vi "模拟量输入自动测试一组_fast_OK.vi"(8 "AD选择？":bool, 9 "DSP选择？":bool, 11 "第几个":i32) -> ()   [LabVIEW 2010]
uses:
  全局量/试验配置信息.vi
panel:
  in  "AD测试值":dbl[](array[numeric])
  in  "DSP测试值":dbl[](array[numeric])
  # "从0开始"
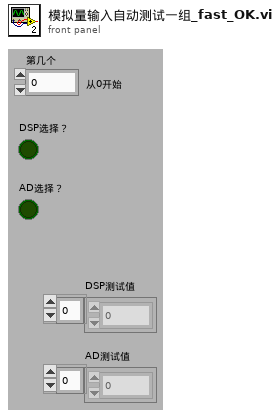
[diagram p1: front panel]
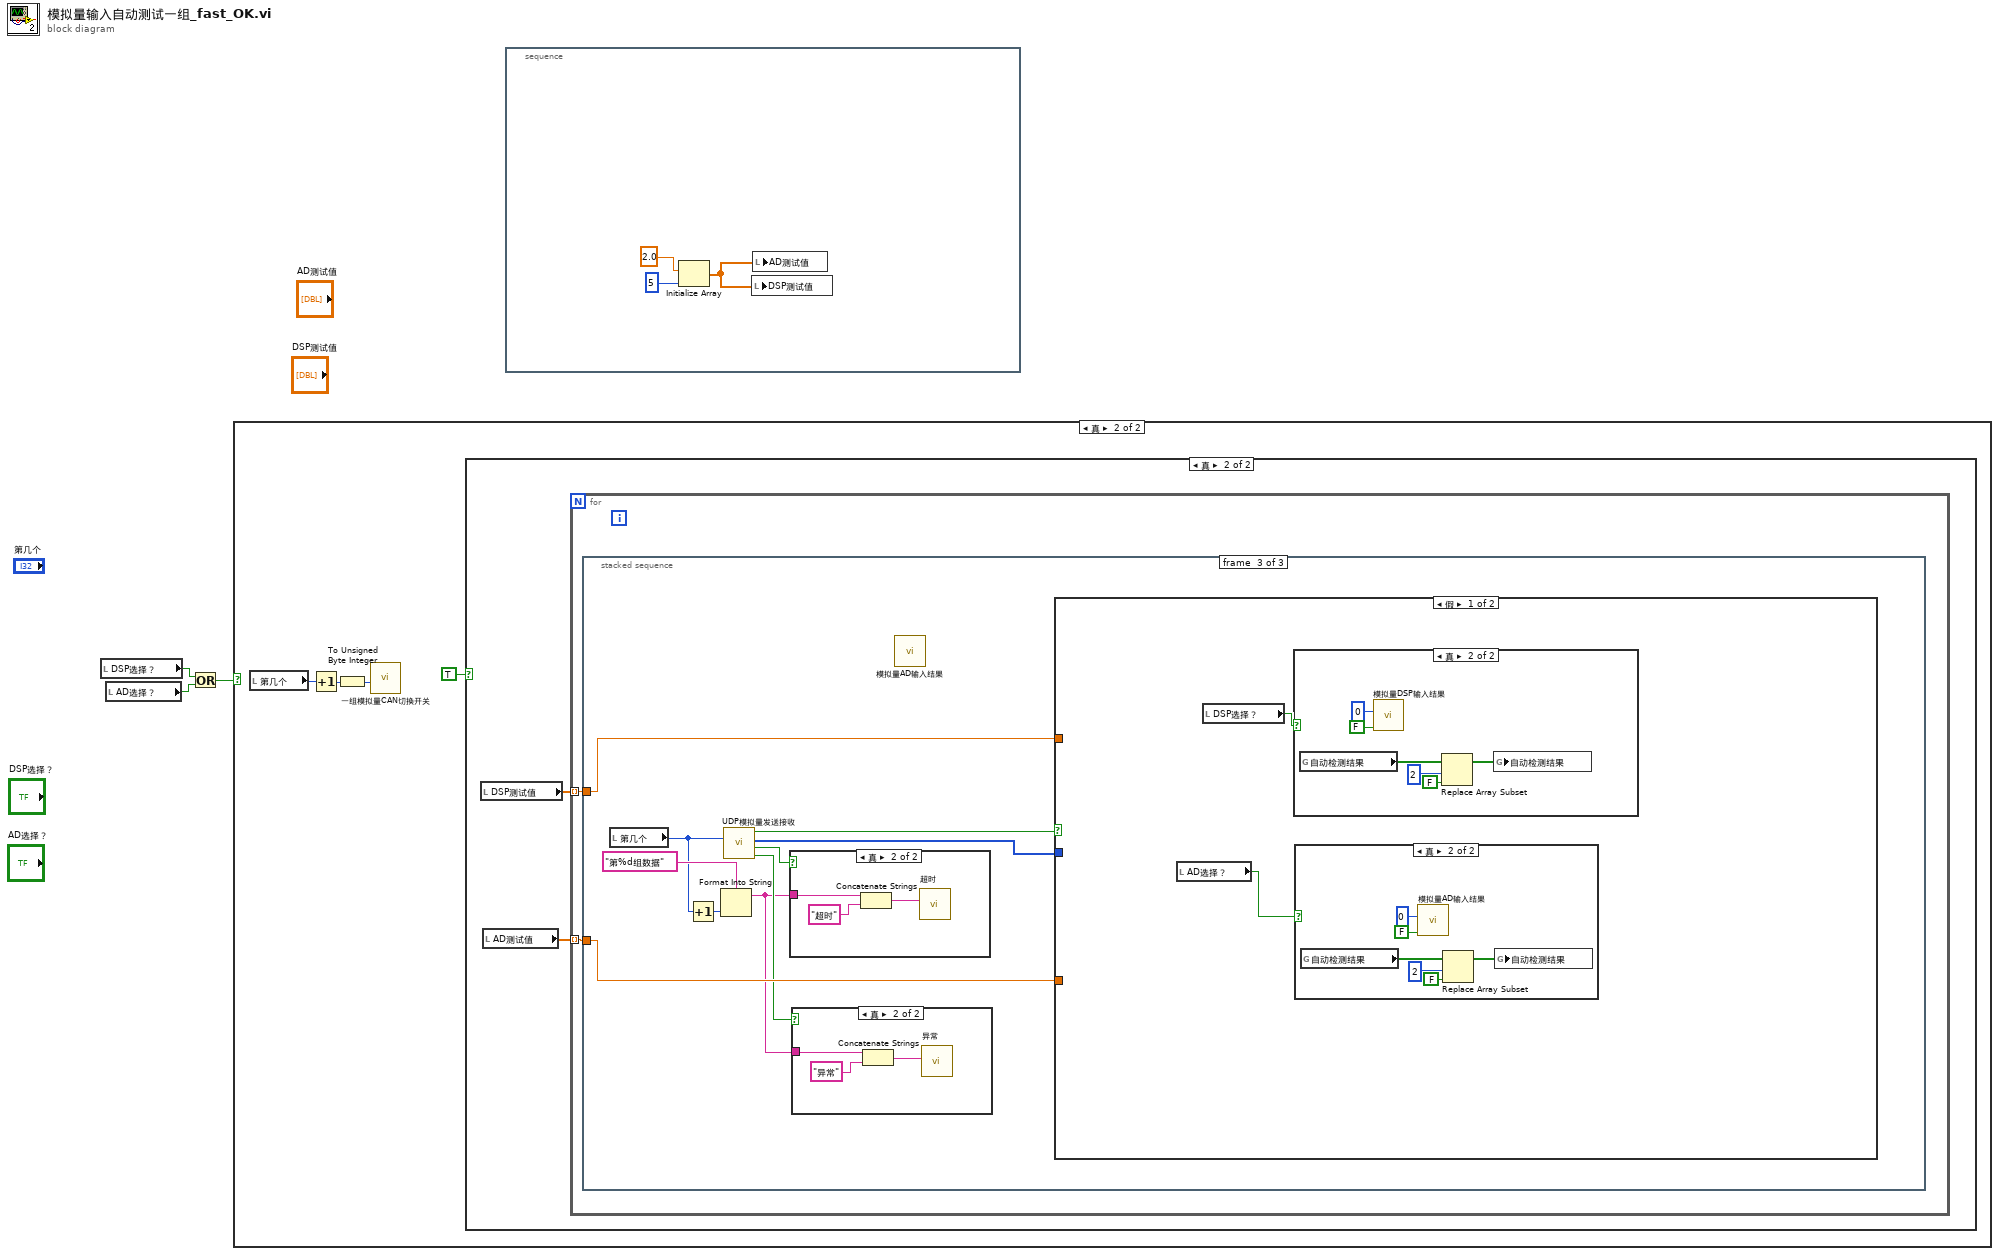
[diagram p0: block diagram]
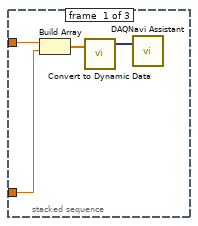
[diagram p4: hidden frame]
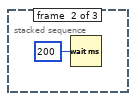
[diagram p5: hidden frame]
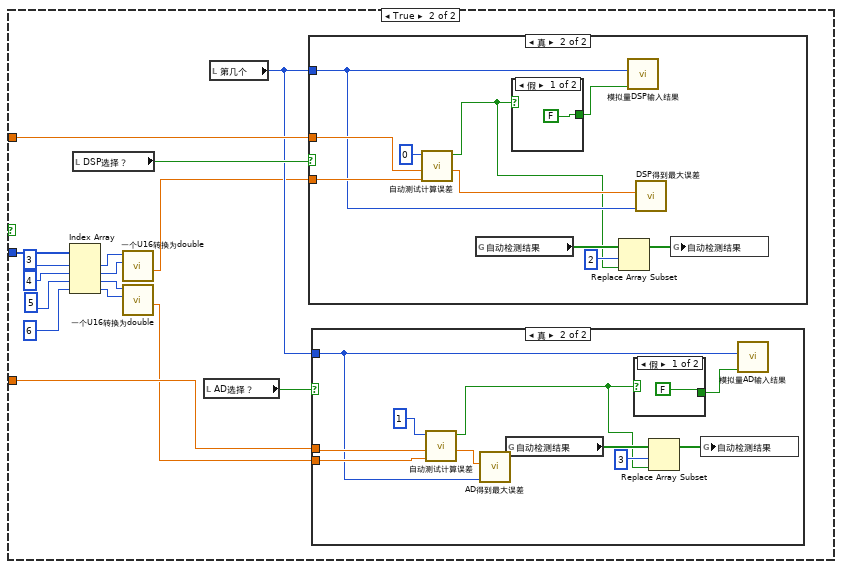
[diagram p10: hidden frame]
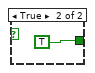
[diagram p12: hidden frame]
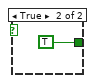
[diagram p14: hidden frame]
diagram:
  n1 = local read "DSP选择？"() -> (w2:bool)
  n2 = local read "AD选择？"() -> (w3:bool)
  n3 = Or(x=w2, y=w3) -> (x .or. y?=w1:bool)
  n4 = case shown="真" w1 {
    frame False {
    }
    frame True {
      n5 = local read "第几个"() -> (w7:i32)
      n6 = Increment(x=w7) -> (x+1=w5:i32)
      n7 = To Unsigned Byte Integer(number=w5) -> (unsigned 8bit integer=w6:u8)
      n8 = call "一组模拟量CAN切换开关.vi"("第几组数据"=w6) -> ()  [unwired: 10 in, 1 out]
      n9 = case shown="真" TRUE {
        frame False {
        }
        frame True {
          n10 = local read "DSP测试值"() -> (w9:dbl[])
          n11 = local read "AD测试值"() -> (w8:dbl[])
          n12 = for {
            tunnel: w9 -> [w11] mode=indexing
            tunnel: w8 -> [w10] mode=indexing
            n13 = stacked-sequence {
              tunnel: w11 -> [w13 _ w26]
              tunnel: w10 -> [w12 _ w25]
              frame #0 {
                n14 = Build Array(w13, w12) -> (w15:dbl[])
                n15 = call "Convert to Dynamic Data"("Array"=w15) -> ("Dynamic Data Type"=w14:dynamicdata)  [unwired: 3 out]
                n16 = call "DAQNavi Assistant"("data in(DDT)"=w14) -> ()  [unwired: 2 in, 17 out]
              }
              frame #1 {
                n17 = Wait (ms)(milliseconds to wait=u32 200 ("等待时间（毫秒）")) -> ()  [unwired: 1 out]
              }
              frame #2 {
                n18 = local read "第几个"() -> (w18:i32)
                n19 = Increment(x=w18) -> (x+1=w19:i32)
                n20 = Format Into String(format string="第%d组数据" ("格式字符串"), w19) -> (resulting string=w20:string)  [unwired: 2 in, 1 out]
                n21 = call "UDP模拟量发送接收.vi"("第几组"=w18) -> ("异常_找到?"=w21:bool, "接收超时?"=w17:bool, "接收的一帧数据"=w24:u16[], "正常_找到?"=w23:bool)  [unwired: 7 in]
                n22 = case shown="真" w17 {
                  tunnel: w20 -> [_ w32]
                  frame False {
                  }
                  frame True {
                    n23 = Concatenate Strings(w32, "超时" ("格式字符串")) -> (w30:string)
                    n24 = call "超时"("Message"=w30) -> ()  [unwired: 9 in, 2 out]
                  }
                }
                n25 = case shown="真" w21 {
                  tunnel: w20 -> [_ w29]
                  frame False {
                  }
                  frame True {
                    n26 = Concatenate Strings(w29, "异常" ("格式字符串")) -> (w27:string)
                    n27 = call "异常"("Message"=w27) -> ()  [unwired: 9 in, 2 out]
                  }
                }
                n28 = call "模拟量AD输入结果.vi"() -> ()  [unwired: 12 in]
                n29 = case shown="假" w23 {
                  tunnel: w24 -> [_ w54]
                  tunnel: w26 -> [_ w52]
                  tunnel: w25 -> [_ w51]
                  frame False {
                    n30 = local read "AD选择？"() -> (w33:bool)
                    n31 = local read "DSP选择？"() -> (w34:bool)
                    n32 = case shown="真" w34 {
                      frame False {
                      }
                      frame True {
                        n33 = global read "试验配置信息.vi" "自动检测结果"() -> (w42:bool[])
                        n34 = call "模拟量DSP输入结果.vi"("合格?"=FALSE, "第几个"=0) -> ()  [unwired: 10 in]
                        n35 = Replace Array Subset(array=w42, new element=FALSE ("新元素/子数组"), index=2 ("索引")) -> (w43:bool[])
                        n36 = global write "试验配置信息.vi" "自动检测结果"(w43) -> ()
                      }
                    }
                    n37 = case shown="真" w33 {
                      frame False {
                      }
                      frame True {
                        n38 = global read "试验配置信息.vi" "自动检测结果"() -> (w38:bool[])
                        n39 = call "模拟量AD输入结果.vi"("合格?"=FALSE, "第几个"=0) -> ()  [unwired: 10 in]
                        n40 = Replace Array Subset(array=w38, new element=FALSE ("新元素/子数组"), index=2 ("索引")) -> (w37:bool[])
                        n41 = global write "试验配置信息.vi" "自动检测结果"(w37) -> ()
                      }
                    }
                  }
                  frame True {
                    n42 = Index Array(array=w54, index #1=3 ("索引"), index #2=4 ("索引"), index #3=5 ("索引"), index #4=6 ("索引")) -> (element #1=w59:u16, element #2=w60:u16, element #3=w61:u16, element #4=w62:u16)
                    n43 = local read "DSP选择？"() -> (w53:bool)
                    n44 = call "一个U16转换为double.vi"("低16位_1"=w60, "高16位_1"=w59) -> ("反馈值"=w47:dbl)  [unwired: 9 in]
                    n45 = call "一个U16转换为double.vi"("低16位_1"=w62, "高16位_1"=w61) -> ("反馈值"=w50:dbl)  [unwired: 9 in]
                    n46 = local read "AD选择？"() -> (w49:bool)
                    n47 = local read "第几个"() -> (w48:i32)
                    n48 = case shown="真" w53 {
                      tunnel: w52 -> [_ w83]
                      tunnel: w47 -> [_ w82]
                      tunnel: w48 -> [_ w79]
                      frame False {
                      }
                      frame True {
                        n49 = call "自动测试计算误差.vi"("反馈值"=w82, "输入值"=w83, "DSP_OR_AD"=0) -> ("误差"=w80:dbl, "合格？"=w75:bool)  [unwired: 7 in]
                        n50 = global read "试验配置信息.vi" "自动检测结果"() -> (w76:bool[])
                        n51 = case shown="假" w75 {
                          tunnel: [FALSE TRUE] -> w81
                          frame False {
                          }
                          frame True {
                          }
                        }
                        n52 = Replace Array Subset(array=w76, new element=w75, index=2 ("索引")) -> (w77:bool[])
                        n53 = call "模拟量DSP输入结果.vi"("合格?"=w81, "第几个"=w79) -> ()  [unwired: 10 in]
                        n54 = call "DSP得到最大误差.vi"("第几组"=w79, "新误差值"=w80) -> ()  [unwired: 10 in]
                        n55 = global write "试验配置信息.vi" "自动检测结果"(w77) -> ()
                      }
                    }
                    n56 = case shown="真" w49 {
                      tunnel: w51 -> [_ w71]
                      tunnel: w50 -> [_ w70]
                      tunnel: w48 -> [_ w67]
                      frame False {
                      }
                      frame True {
                        n57 = call "自动测试计算误差.vi"("反馈值"=w70, "输入值"=w71, "DSP_OR_AD"=1) -> ("误差"=w68:dbl, "合格？"=w63:bool)  [unwired: 7 in]
                        n58 = call "AD得到最大误差.vi"("第几组"=w67, "新误差值"=w68) -> ()  [unwired: 10 in]
                        n59 = global read "试验配置信息.vi" "自动检测结果"() -> (w66:bool[])
                        n60 = case shown="假" w63 {
                          tunnel: [FALSE TRUE] -> w69
                          frame False {
                          }
                          frame True {
                          }
                        }
                        n61 = Replace Array Subset(array=w66, new element=w63, index=3 ("索引")) -> (w65:bool[])
                        n62 = global write "试验配置信息.vi" "自动检测结果"(w65) -> ()
                        n63 = call "模拟量AD输入结果.vi"("合格?"=w69, "第几个"=w67) -> ()  [unwired: 10 in]
                      }
                    }
                  }
                }
              }
            }
          }
        }
      }
    }
  }
  n64 = stacked-sequence {
    frame #0 {
      n65 = Initialize Array(2.0, 5 ("维数大小")) -> (w87:dbl[])
      n66 = local write "DSP测试值"(w87) -> ()
      n67 = local write "AD测试值"(w87) -> ()
    }
  }
